vi "ClosePort.vi"   [LabVIEW 2017]
uses:
  <vilib>/Instr/_visa.llb/VISA Find Search Mode.ctl
types:
  T1 = typedef "VISA Find Search Mode.ctl" = u32
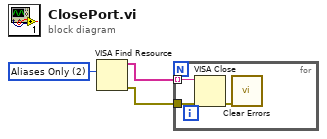
[diagram p0: block diagram]
diagram:
  w3 = T1 2 items=["Canonical Names Only"=0, "Aliases Only"=2, "Include Matching Aliases"=3, "Include All Aliases"=4] ("Search Mode")
  n1 = VISA Find Resource(10:w3) -> (0:w1:errorcluster, 3:w2:string[])  [unwired: 2 in, 1 out]
  n2 = for {
    tunnel: w2 -> [w5] mode=indexing
    tunnel: w1 -> [w4]
    n3 = VISA Close(VISA resource name=w5, error in (no error)=w4) -> (error out=w6:errorcluster)
    n4 = call <vilib>:"Clear Errors.vi"("error in (no error)"=w6) -> ()  [unwired: 5 in, 2 out]
  }
